vi "Read Image Strips.vi"(8 "First Strip":u32, 10 "Column IN":i16[](array[numeric]), 11 "DATA IN":u8[](array[numeric])) -> (0 "Next Strip":u32, 1 "Enf of Column?":bool, 2 "Column OUT":i16[](array[numeric]))   [LabVIEW 2017]
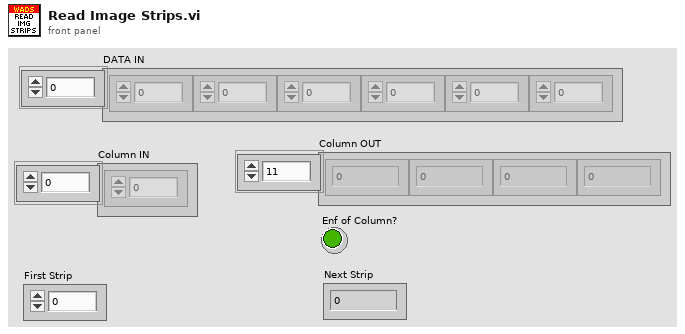
[diagram p1: front panel]
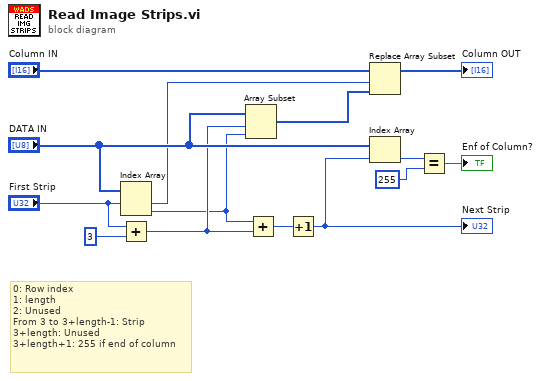
[diagram p0: block diagram]
diagram:
  # "0: Row index\n1: length\n2: Unused\nFrom 3 to 3+length-1: Strip\n3+length: Unused\n3+length+1: 255 if end of column"
  n1 = Index Array(array="DATA IN", index #1="First Strip") -> (element #1=w8:u8, element #2=w11:u8)  [unwired: 1 in]
  n2 = Add(x="First Strip", y=3) -> (x+y=w12:u32)
  n3 = Array Subset(array="DATA IN", index=w12, length=w11) -> (w9:u8[])
  n4 = Add(x=w11, y=w12) -> (x+y=w14:u32)
  n5 = Increment(x=w14) -> (x+1=w1:u32)
  "Next Strip" <- w1
  n6 = Replace Array Subset(array="Column IN", new element=w9, index=w8) -> (→"Column OUT":i16[])
  n7 = Index Array(array="DATA IN", index=w1) -> (element=w4:u8)
  n8 = Equal?(x=w4, y=255) -> (x = y?=→"Enf of Column?":bool)
